vi "CRYSet Channel Changing State.vi"(8 "Name In":string[][](array[string]), 9 "New Channel Name":string, 10 "Old Channel Name":string, 11 "Mode":enum16{"Add", "Delete", "Rename", "Load/Revert"}(ring)) -> (0 "Name Out":string[][](array[string]))   [LabVIEW 2013]
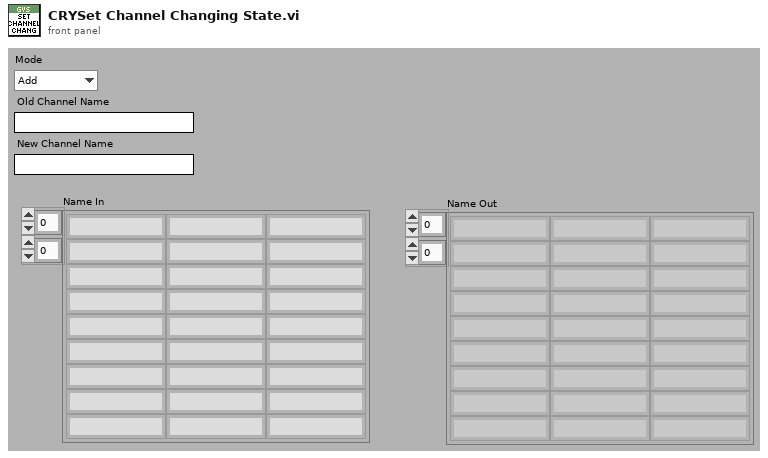
[diagram p1: front panel]
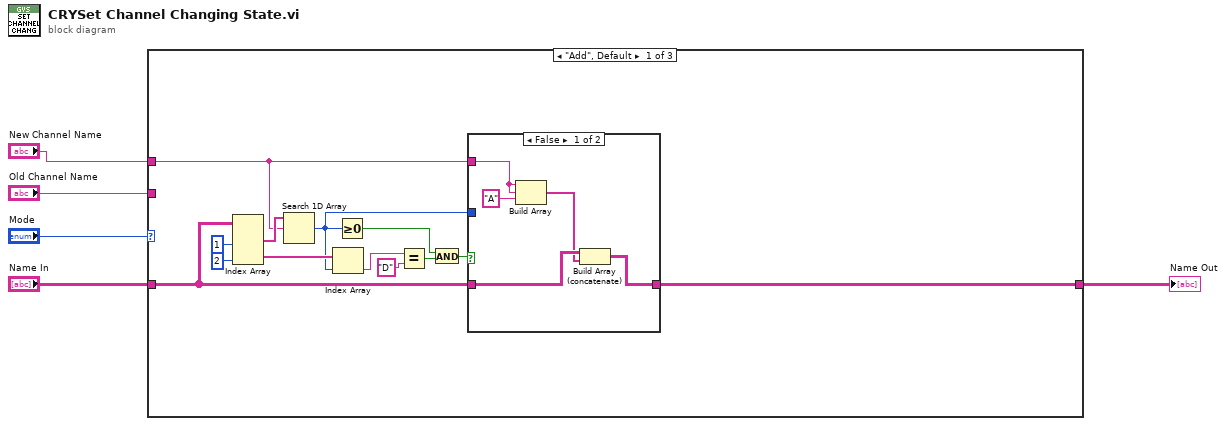
[diagram p0: block diagram]
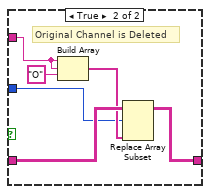
[diagram p2: hidden frame]
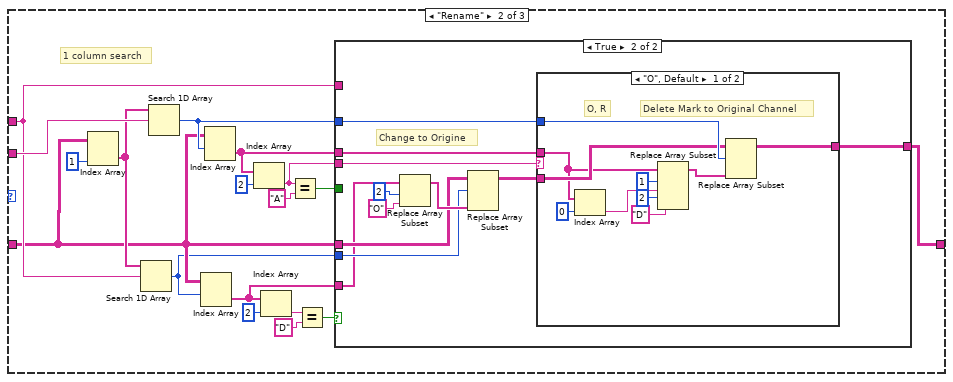
[diagram p3: hidden frame]
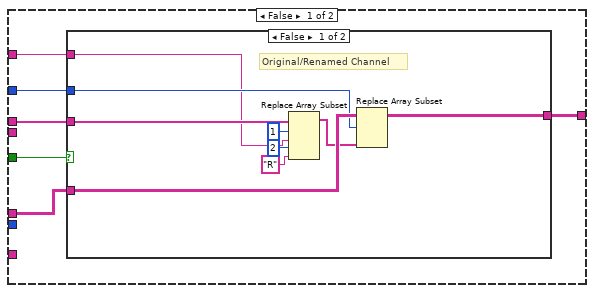
[diagram p4: hidden frame]
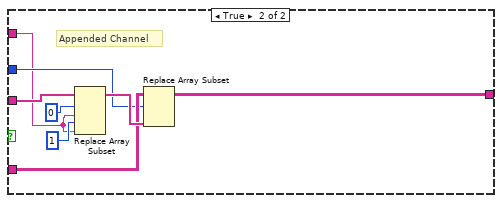
[diagram p5: hidden frame]
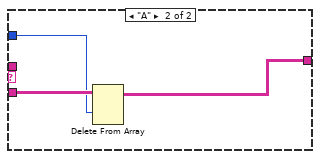
[diagram p6: hidden frame]
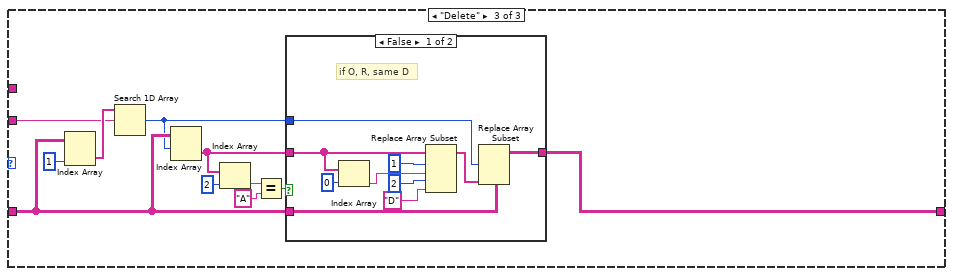
[diagram p7: hidden frame]
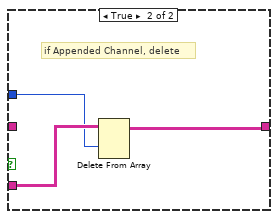
[diagram p8: hidden frame]
diagram:
  n1 = case shown="\"Add\", Default" "Mode" {
    tunnel: "Name In" -> [w16 w37 w102]
    tunnel: [w18 w40 w100] -> w3
    tunnel: "New Channel Name" -> [w7 w39 _]
    tunnel: "Old Channel Name" -> [_ w44 w103]
    frame "Add", Default {
      n2 = Index Array(array=w16, index (col) #1=1 ("disabled index (col)"), index (col) #2=2 ("index (col)")) -> (element #1=w15:string[], element #2=w13:string[])  [unwired: 2 in]
      n3 = Search 1D Array(1D array=w15, element=w7) -> (index of element=w6:i32)  [unwired: 1 in]
      n4 = Index Array(array=w13, index=w6) -> (element=w12:string)
      n5 = Greater Or Equal To 0?(x=w6) -> (x >= 0?=w9:bool)
      n6 = Equal?(x=w12, y="D") -> (x = y?=w10:bool)
      n7 = And(x=w9, y=w10) -> (x .and. y?=w8:bool)
      n8 = case shown="False" w8 {
        tunnel: [w23 w24] -> w18
        tunnel: w16 -> [w22 w27]
        tunnel: w7 -> [w20 w28]
        tunnel: w6 -> [_ w25]
        frame False {
          n9 = Build Array(w20, w20, "A" ("element")) -> (w19:string[])
          n10 = Build Array (concatenate)(w22, w19) -> (w23:string[][])
        }
        frame True {
          # "Original Channel is Deleted"
          n11 = Build Array(w28, w28, "O" ("element")) -> (w26:string[])
          n12 = Replace Array Subset(array=w27, new element=w26, index (row)=w25) -> (w24:string[][])  [unwired: 1 in]
        }
      }
    }
    frame "Rename" {
      # "1 column search"
      n13 = Index Array(array=w37, index (col)=1 ("disabled index (col)")) -> (element=w38:string[])  [unwired: 1 in]
      n14 = Search 1D Array(1D array=w38, element=w39) -> (index of element=w32:i32)  [unwired: 1 in]
      n15 = Search 1D Array(1D array=w38, element=w44) -> (index of element=w41:i32)  [unwired: 1 in]
      n16 = Index Array(array=w37, index (row)=w32) -> (element=w31:string[])  [unwired: 1 in]
      n17 = Index Array(array=w37, index (row)=w41) -> (element=w42:string[])  [unwired: 1 in]
      n18 = Index Array(array=w42, index=2) -> (element=w30:string)
      n19 = Index Array(array=w31, index=2) -> (element=w35:string)
      n20 = Equal?(x=w30, y="A") -> (x = y?=w43:bool)
      n21 = Equal?(x=w35, y="D") -> (x = y?=w33:bool)
      n22 = case shown="True" w33 {
        tunnel: w43 -> [w53 _]
        tunnel: w42 -> [w52 w71]
        tunnel: w41 -> [w51 w73]
        tunnel: [w50 w72] -> w40
        tunnel: w39 -> [w49 _]
        tunnel: w37 -> [w48 w80]
        tunnel: w32 -> [_ w79]
        tunnel: w31 -> [_ w76]
        tunnel: w30 -> [_ w75]
        frame False {
          n23 = case shown="False" w53 {
            tunnel: w48 -> [w62 w68]
            tunnel: [w61 w67] -> w50
            tunnel: w52 -> [w59 w66]
            tunnel: w51 -> [w60 w65]
            tunnel: w49 -> [w57 w63]
            frame False {
              # "Original/Renamed Channel"
              n24 = Replace Array Subset(array=w59, new element #1=w57, index #1=1 ("index"), new element #2="R" ("new element/subarray"), index #2=2 ("index")) -> (w54:string[])
              n25 = Replace Array Subset(array=w62, new element=w54, index (row)=w60) -> (w61:string[][])  [unwired: 1 in]
            }
            frame True {
              # "Appended Channel"
              n26 = Replace Array Subset(array=w66, new element #1=w63, index #1=0 ("index"), new element #2=w63, index #2=1 ("index")) -> (w69:string[])
              n27 = Replace Array Subset(array=w68, new element=w69, index (row)=w65) -> (w67:string[][])  [unwired: 1 in]
            }
          }
        }
        frame True {
          # "Change to Origine"
          n28 = Replace Array Subset(array=w76, new element="O" ("new element/subarray"), index=2) -> (w81:string[])
          n29 = Replace Array Subset(array=w80, new element=w81, index (row)=w79) -> (w74:string[][])  [unwired: 1 in]
          n30 = case shown="\"O\", Default" w75 {
            tunnel: w74 -> [w85 w94]
            tunnel: w73 -> [w87 w93]
            tunnel: [w88 w92] -> w72
            tunnel: w71 -> [w84 _]
            frame "O", Default {
              # "Delete Mark to Original Channel"
              # "O, R"
              n31 = Index Array(array=w84, index=0) -> (element=w83:string)
              n32 = Replace Array Subset(array=w84, new element #1=w83, index #1=1 ("index"), new element #2="D" ("new element/subarray"), index #2=2 ("index")) -> (w89:string[])
              n33 = Replace Array Subset(array=w85, new element=w89, index (row)=w87) -> (w88:string[][])  [unwired: 1 in]
            }
            frame "A" {
              n34 = Delete From Array(array=w94, index (row)=w93) -> (array with subset deleted=w92:string[][])  [unwired: 2 in, 1 out]
            }
          }
        }
      }
    }
    frame "Delete" {
      n35 = Index Array(array=w102, index (col)=1 ("disabled index (col)")) -> (element=w104:string[])  [unwired: 1 in]
      n36 = Search 1D Array(1D array=w104, element=w103) -> (index of element=w101:i32)  [unwired: 1 in]
      n37 = Index Array(array=w102, index (row)=w101) -> (element=w99:string[])  [unwired: 1 in]
      n38 = Index Array(array=w99, index=2) -> (element=w97:string)
      n39 = Equal?(x=w97, y="A") -> (x = y?=w95:bool)
      n40 = case shown="False" w95 {
        tunnel: w102 -> [w115 w118]
        tunnel: w101 -> [w114 w117]
        tunnel: [w113 w116] -> w100
        tunnel: w99 -> [w108 _]
        frame False {
          # "if O, R, same D"
          n41 = Index Array(array=w108, index=0) -> (element=w106:string)
          n42 = Replace Array Subset(array=w108, new element #1=w106, index #1=1 ("index"), new element #2="D" ("new element/subarray"), index #2=2 ("index")) -> (w112:string[])
          n43 = Replace Array Subset(array=w115, new element=w112, index (row)=w114) -> (w113:string[][])  [unwired: 1 in]
        }
        frame True {
          # "if Appended Channel, delete"
          n44 = Delete From Array(array=w118, index (row)=w117) -> (array with subset deleted=w116:string[][])  [unwired: 2 in, 1 out]
        }
      }
    }
  }
  "Name Out" <- w3
